vi "get position.vi"(8 "error in (no error)":errorcluster, 10 "the_get_position":T1, 11 "id":i32) -> (0 "error out":errorcluster, 2 "the_get_position out":T1, 3 "function return":i32)   [LabVIEW 2012, in "libximc.lvlib"]
doc: "result_t XIMC_API get_position (device_t id, get_position_t* the_get_position);"
uses:
  libximc.lvlib
  libximc.dll
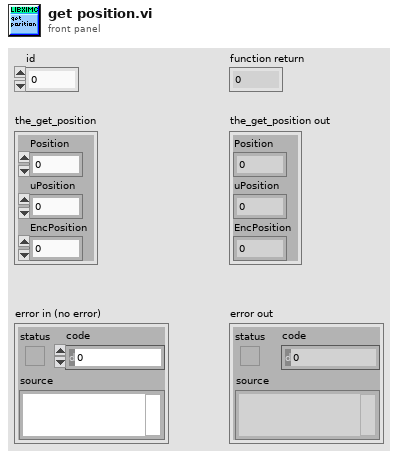
[diagram p1: front panel]
types:
  T1 = cluster{"Position":i32, "uPosition":i32, "EncPosition":i64}
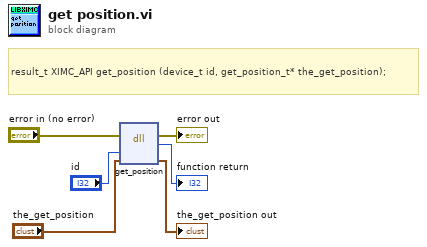
[diagram p0: block diagram]
diagram:
  # "result_t XIMC_API get_position (device_t id, get_position_t* the_get_position);"
  n1 = dll-call lib="C:/Users/Stepan/Downloads/labview_2.9.11_testgen_thread/libximc.*" fn="get_position"(error in="error in (no error)", "id"="id", "the_get_position"="the_get_position") -> (error out=→"error out":errorcluster, →"function return":i32, "the_get_position"=→"the_get_position out":T1)  [unwired: 3 in, 1 out]
